vi "Launcher.vi"   [LabVIEW 2023]
uses:
  [MV] Key Certify/[MV] Key Certify/[MV] Key Certify.lvclass
  C:/Program Files (x86)/National Instruments/LabVIEW 2023/vi.lib/ActorFramework/Actor/Actor.lvclass
  <vilib>/ActorFramework/Actor/Actor.lvclass
  [MV] Key Certify/[MV] Key Certify/[MV] Key Certify.lvclass/[MV] Key Certify.ctl
  [MV] Key Certify/[MV] Key Certify/Accessor/Write actor.vi
  [MV] Key Certify/[MV] Key Certify/Accessor/Write key folder.vi
  [MV] Key Certify/[MV] Key Certify/Accessor/Write public key.vi
  [MV] Key Certify/[MV] Key Certify/Accessor/Write software name.vi
panel:
  # "激活"
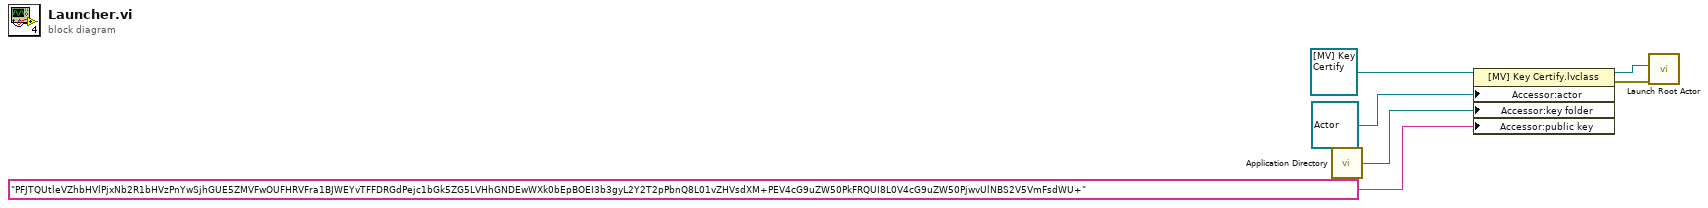
[diagram p0: block diagram]
diagram:
  n1 = call <vilib>:"Application Directory.vi"() -> ("Application Directory"=w5:path)
  n2 = property class="[MV] Key Certify.lvclass"(reference=refnum<class "[MV] Key Certify.lvclass"> refnum ("[MV] Key Certify.lvlib:[MV] Key Certify.lvclass"), "Accessor:actor"=refnum<class "Actor.lvclass"> refnum ("actor"), "Accessor:key folder"=w5, "Accessor:public key"="PFJTQUtleVZhbHVlPjxNb2R1bHVzPnYwSjhGUE5ZMVFwOUFHRVFra1BJWEYvTFFDRGdPejc1bGk5ZG5LVHhGNDEwWXk0bEpBOEI3b3gyL2Y2T2pPbnQ8L01vZHVsdXM+PEV4cG9uZW50PkFRQUI8L0V4cG9uZW50PjwvUlNBS2V5VmFsdWU+" ("public key")) -> (reference out=w1:refnum<class "[MV] Key Certify.lvclass">, error out=w2:errorcluster)  [unwired: 1 in]
  n3 = call <vilib>:"Launch Root Actor.vi"("error in (no error)"=w2, "Actor"=w1) -> ()  [unwired: 8 in, 2 out]
